vi "Read Camera Snapshot.vi"(0 "image in":refnum<class "MSC Image.lvclass">, 1 "camID":i32, 5 "error in (no error)":errorcluster) -> (14 "image out":refnum<class "MSC Image.lvclass">, 19 "error out":errorcluster)   [LabVIEW 2014, in "MSC Image.lvclass"]
doc: "Simple method for capuring a frame from a camera. Use the ID to switch between cameras.\n\nSupported drivers are:\nMIL, VFW, V4L, V4L2, Fireware, Firewire, IEEE 1394, DC, Stereo TYZX, Quicktime, Unicap, DirectShow, PvAPI, Prosilica GigE, OpenNI, XIMEA Camera"
uses:
  MSC Image.lvclass
  MSC Image.lvclass/MSC Image.ctl
  Dependencies/x86/MSC I Process32.dll
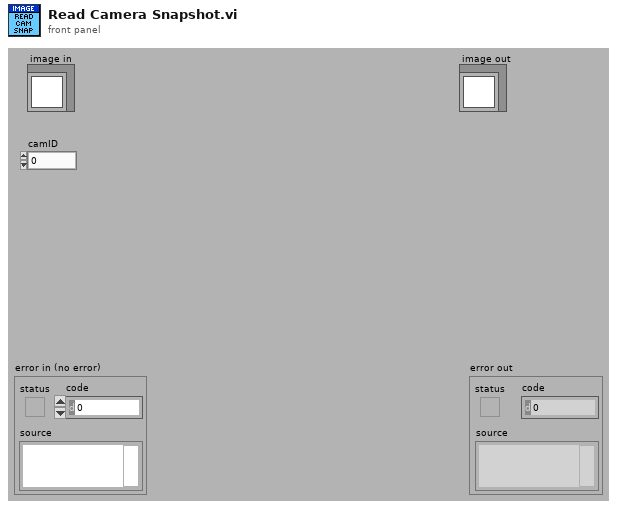
[diagram p1: front panel]
types:
  T1 = typedef "Image.ctl" = cluster{"Pointer":u64, "Size":T2, "Image Type":T3, "Time Stamp":timestamp, "Variant":variant}
  T2 = typedef "Size.ctl" = cluster{"Cols":i32, "Rows":i32}
  T3 = typedef "Image Type.ctl" = i32
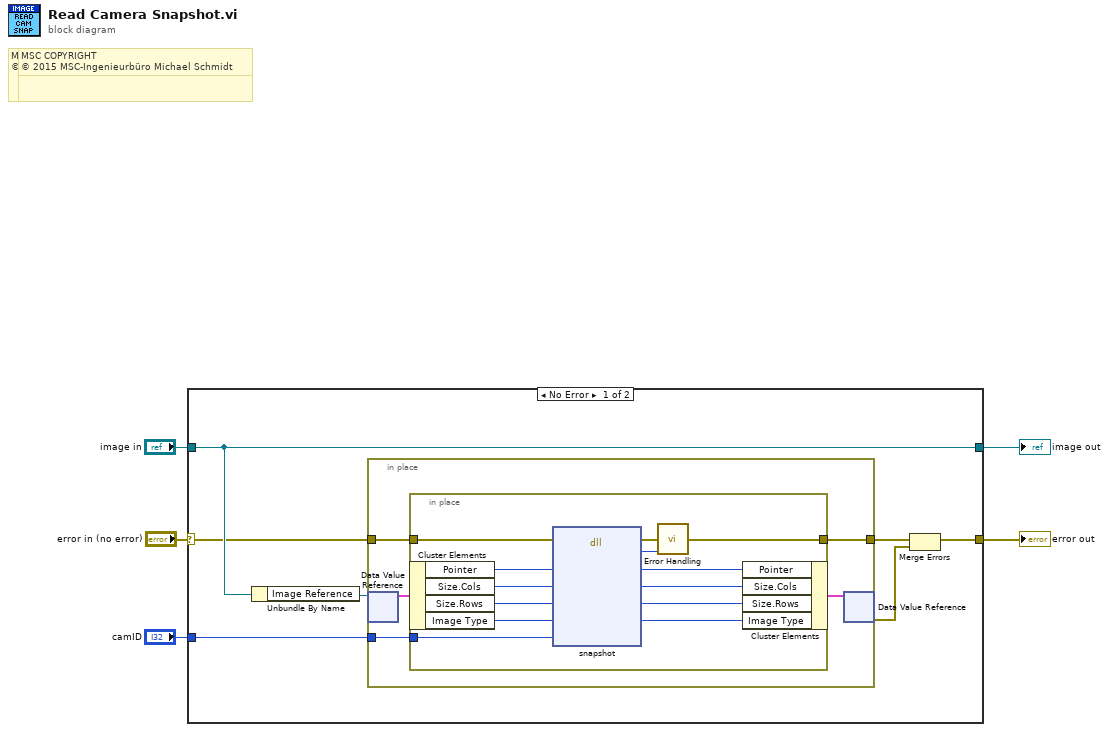
[diagram p0: block diagram]
diagram:
  # "MSC COPYRIGHT\n© 2016 MSC-Ingenieurbüro Michael Schmidt"
  # "MSC COPYRIGHT\n© 2016 MSC-Ingenieurbüro Michael Schmidt"
  # "MSC COPYRIGHT\n© 2015 MSC-Ingenieurbüro Michael Schmidt"
  # "MSC COPYRIGHT\n© 2015 MSC-Ingenieurbüro Michael Schmidt"
  n1 = case shown="No Error" "error in (no error)" {
    selector: "error in (no error)" -> [w8 w32]
    tunnel: [w7 w32] -> w4
    tunnel: [w12 w31] -> w2
    tunnel: "image in" -> [w12 w31]
    tunnel: "camID" -> [w6 _]
    frame No Error {
      n2 = Unbundle By Name(w12) -> ("Image Reference"=w11:refnum<data-value>)
      n3 = in-place {
        in-place-border: w8 -> [w15]
        in-place-border: [w14] -> w10
        in-place-border: w6 -> [w13]
        n4 = in-place-dvr #1(w11) -> (w16:T1)  [unwired: 1 out]
        n5 = in-place {
          in-place-border: w15 -> [w19]
          in-place-border: [w25] -> w14
          in-place-border: w13 -> [w18]
          n6 = in-place-cluster #2(w16) -> ("Pointer"=w28:u64, "Size.Cols"=w29:i32, "Size.Rows"=w30:i32, "Image Type"=w22:T3)
          n7 = dll-call lib="C:/Users/MSC/LabVIEW Projekte/LV 2014/MSC I-Process/user.lib/MSC-I Process/Dependencies/x86/MSC I Process*.dll" fn="snapshot"(error in=w19, "pointer"=w28, "cols"=w29, "rows"=w30, "type"=w22, "camID"=w18) -> (error out=w26:errorcluster, "error"=w27:i32, "pointer"=w20:u64, "cols"=w24:i32, "rows"=w23:i32, "type"=w21:i32)  [unwired: 3 in, 1 out]
          n8 = call "Error Handling.vi"("error in (no error)"=w26, "return type"=w27) -> ("error out"=w25:errorcluster)  [unwired: 12 in, 1 out]
          n9 = in-place-cluster #2("Pointer"=w20, "Size.Cols"=w24, "Size.Rows"=w23, "Image Type"=w21) -> (w17:T1)
        }
        n10 = in-place-dvr #1(w17) -> (w9:errorcluster)  [unwired: 1 out]
      }
      n11 = Merge Errors(w10, w9) -> (w7:errorcluster)
    }
    frame Error {
    }
  }
  "error out" <- w4
  "image out" <- w2
